vi "BRig_RT_panel_Laser2_v0,902.vi"(7 "input_setValues":bool, 9 "input_dataExp":u16[](array[numeric]), 11 "input_dataLC":u16[](array[numeric])) -> (1 "output_dataExp":u16[](array[numeric]), 3 "output_dataLC":u16[](array[numeric]))   [LabVIEW 2014]
panel:
  out "LaserPulseTrain":cluster{u16[], u16[]}(graph)
  in  "LED_baseline":bool
  in  "Laser_power_step":dbl
  in  "Laser_power_max":dbl
  in  "Laser_power_min":dbl
  in  "Laser_Tshutter":u16=2
  in  "Laser_Freq":u16=10
  in  "Laser_Tpeak":u16=2
  in  "Laser_T":u16
  in  "LC_Sel_PostR_Count":u16
  in  "LC_Sel_PostR_Probability":u16
  in  "LC_Sel_PostR_Block":u16(slide) max=2 step=1 scale=0.0..2.0
  in  "LC_Sel_PostR_OnOff":bool
  in  "LC_Sel_PostR_Tdelay":u16
  in  "LC_Cue_PostR_Count":u16
  in  "LC_Cue_PostR_delayOpt":bool
  in  "LC_Cue_PostR_Probability":u16
  in  "LC_Cue_PostR_Block":u16(slide) max=2 step=1 scale=0.0..2.0
  in  "LC_Cue_PostR_OnOff":bool
  in  "LC_Cue_PostR_Tdelay":u16
  in  "LC_ENL_PostR_delayOpt":bool
  in  "LC_ENL_PostR_Count":u16
  in  "LC_ENL_PostR_Probability":u16 max=100 step=1
  in  "LC_ENL_PostR_Block":u16(slide) max=2 step=1 scale=0.0..2.0
  in  "LC_ENL_PostR_OnOff":bool
  in  "LC_ENL_PostR_Tdelay":u16
  in  "LC_Sel_PreR_Count":u16
  in  "LC_Sel_First_Count":u16
  in  "LC_Sel_PreR_Probability":u16
  in  "LC_Sel_PreR_Block":u16(slide) max=2 step=1 scale=0.0..2.0
  in  "LC_Sel_PreR_OnOff":bool
  in  "LC_Sel_First_Probability":u16
  in  "LC_Sel_First_Block":u16(slide) max=2 step=1 scale=0.0..2.0
  in  "LC_Sel_First_OnOff":bool
  in  "LC_Sel_PreR_Tdelay":u16
  in  "LC_Sel_First_Tdelay":u16
  in  "LC_Cue_PreR_Count":u16
  in  "LC_Cue_First_Count":u16
  in  "LC_Cue_PreR_delayOpt":bool
  in  "LC_ENL_PreR_delayOpt":bool
  in  "LC_ENL_PreR_Count":u16
  in  "LC_ENL_First_Count":u16
  in  "LC_Cue_First_delayOpt":bool
  in  "LC_ENL_First_delayOpt":bool
  in  "LC_Wrong_Probability":u16
  in  "LC_Wrong_Trial":u16(slide) max=2 step=1 scale=0.0..2.0
  in  "LC_Wrong_Block":u16(slide) max=2 step=1 scale=0.0..2.0
  in  "LC_Wrong_OnOff":bool
  in  "LC_Reward_Probability":u16
  in  "LC_Reward_Trial":u16(slide) max=2 step=1 scale=0.0..2.0
  in  "LC_Reward_Block":u16(slide) max=2 step=1 scale=0.0..2.0
  in  "LC_Reward_OnOff":bool
  in  "LC_Cue_PreR_Probability":u16
  in  "LC_Cue_PreR_Block":u16(slide) max=2 step=1 scale=0.0..2.0
  in  "LC_Cue_PreR_OnOff":bool
  in  "LC_Cue_First_Probability":u16
  in  "LC_Cue_First_Block":u16(slide) max=2 step=1 scale=0.0..2.0
  in  "LC_Cue_First_OnOff":bool
  in  "LC_ENL_PreR_Probability":u16 max=100 step=1
  in  "LC_ENL_PreR_Block":u16(slide) max=2 step=1 scale=0.0..2.0
  in  "LC_ENL_PreR_OnOff":bool
  in  "LC_ENL_First_Probability":u16 max=100 step=1
  in  "LC_ENL_First_Block":u16(slide) max=2 step=1 scale=0.0..2.0
  in  "LC_Wrong_Tdelay":u16
  in  "LC_Cue_PreR_Tdelay":u16
  in  "LC_ENL_PreR_Tdelay":u16
  in  "LC_Reward_Tdelay":u16
  in  "LC_Cue_First_Tdelay":u16
  in  "LC_ENL_First_Tdelay":u16
  in  "LC_ENL_First_OnOff":bool
  # "Laser2 Control\n                               On/Off      Block        Probability [%]   Delay [ms]                              Count"
  # "Enforced\nNonLick"
  # "from end"
  # "First\nTrial"
  # "from start"
  # "from end"
  # "PreReward\nTrials"
  # "from start"
  # "from end"
  # "PostReward\nTrials"
  # "from start"
  # "Cue"
  # "from end"
  # "First\nTrial"
  # "from start"
  # "from end"
  # "PreReward\nTrials"
  # "from start"
  # "from end"
  # "PreReward\nTrials"
  # "from start"
  # "Selection"
  # "from start"
  # "First\nTrial"
  # "from start"
  # "PreReward\nTrials"
  # "from start"
  # "PostReward\nTrials"
  # "Laser2 Parameters"
  # "Laser2 Response\n           On/Off      Block           Trial     Probability %  Delay [ms]"
  # "Frequency\n[Hz]"
  # "Selection\nReward"
  # "Timing [ms]\n Duration     Peak Width   Shutter"
  # "Selection\nWrong"
  # "Laser Power [V]\nMin          Max              Step"
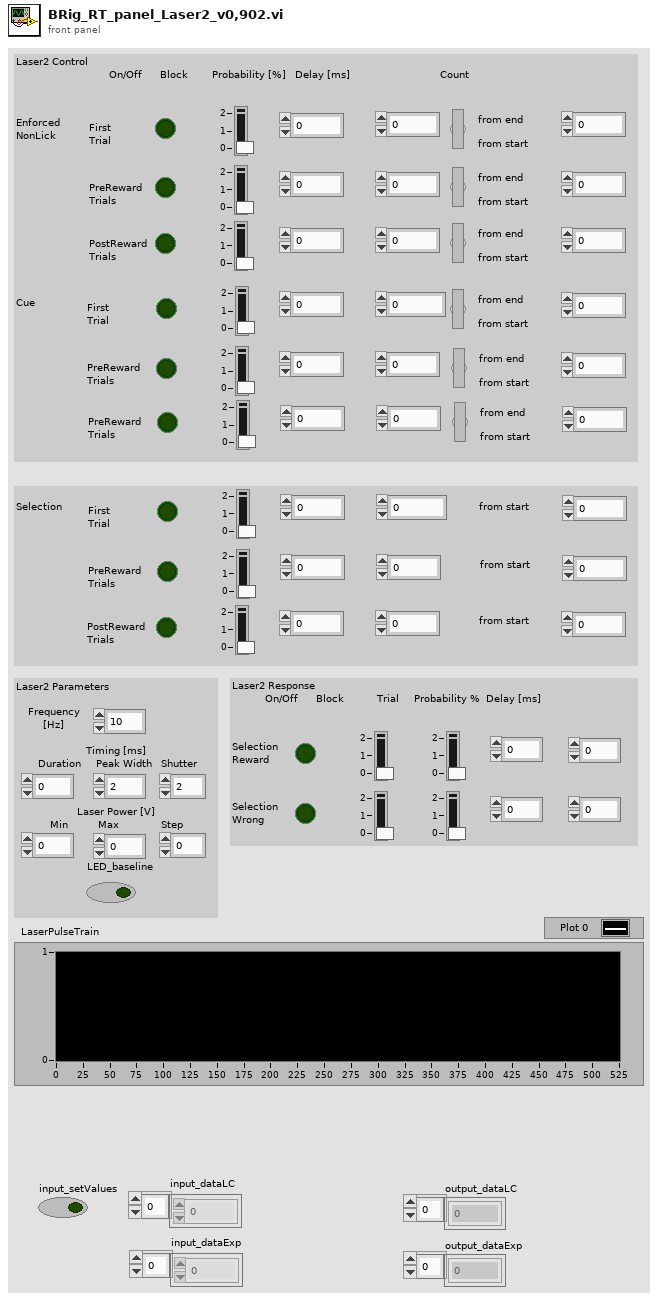
[diagram p1: front panel]
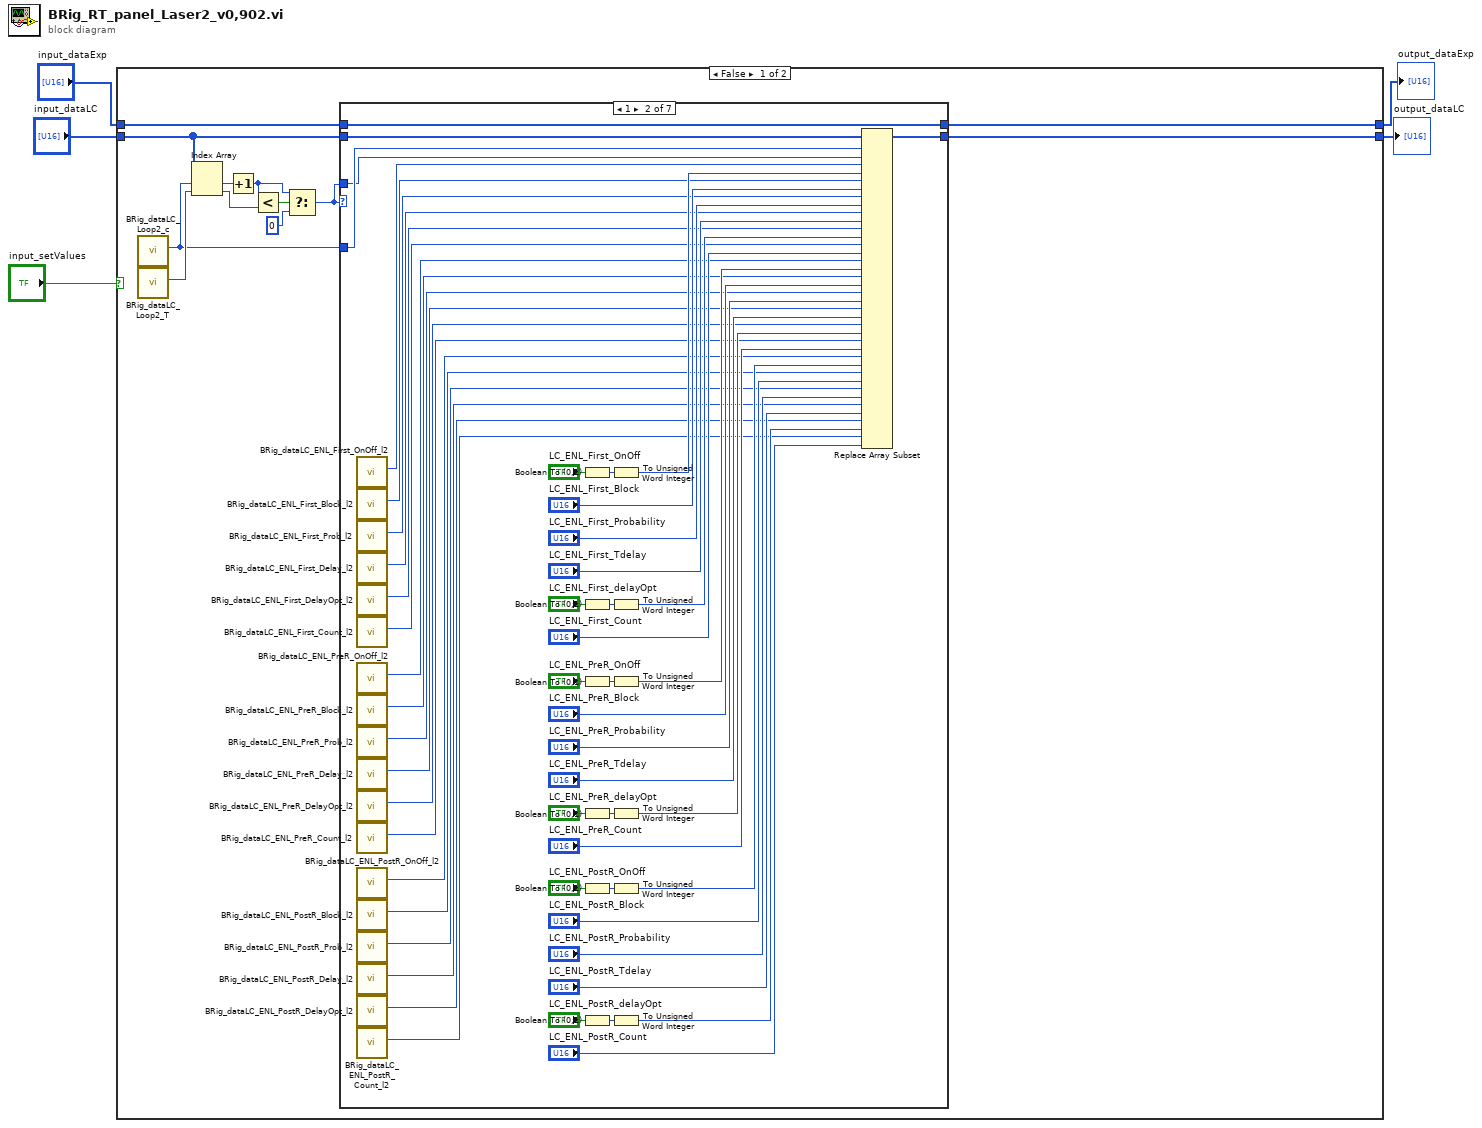
[diagram p0: block diagram]
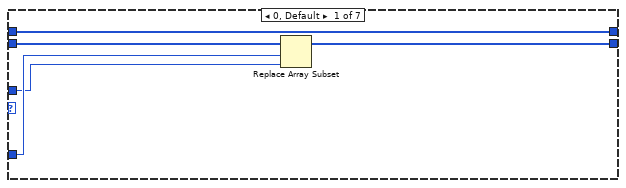
[diagram p2: hidden frame]
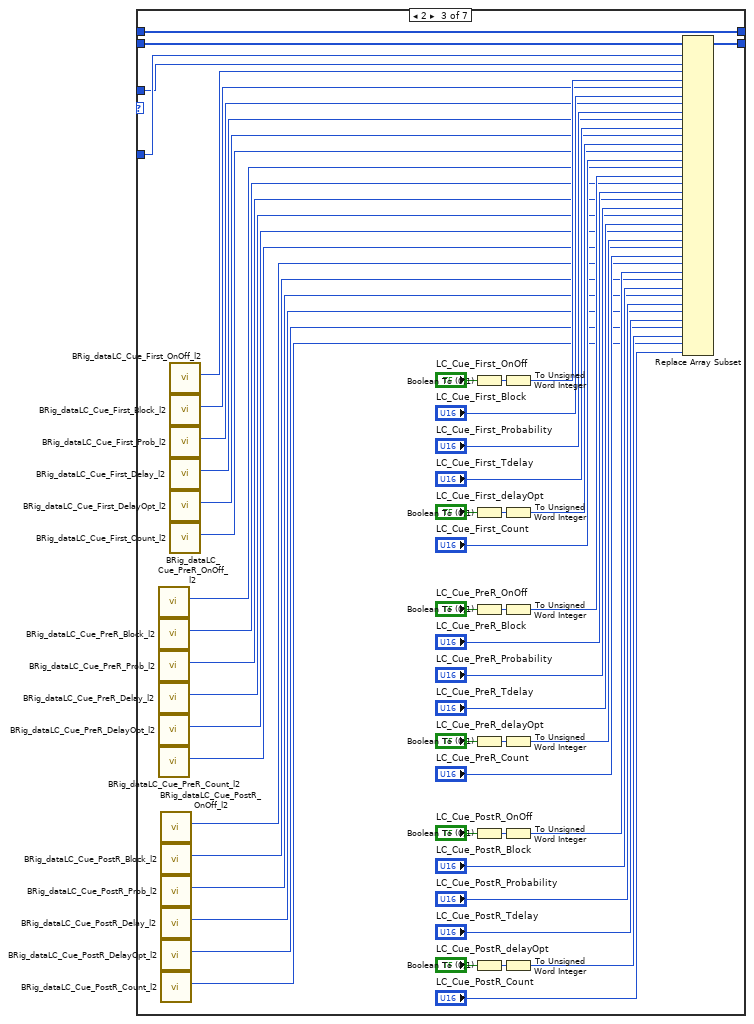
[diagram p3: hidden frame]
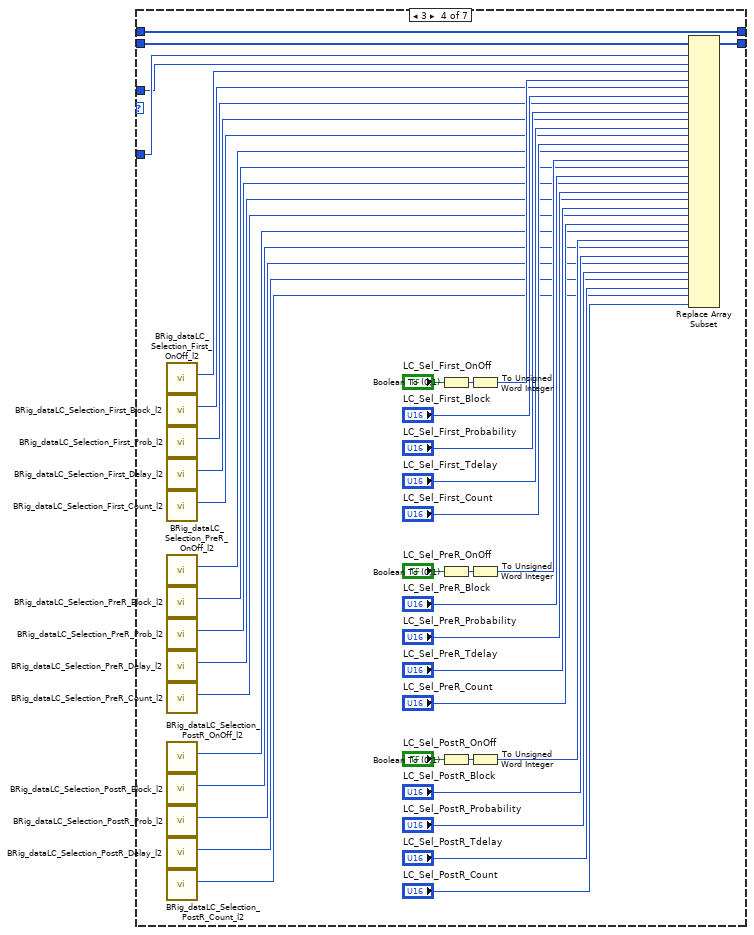
[diagram p4: hidden frame]
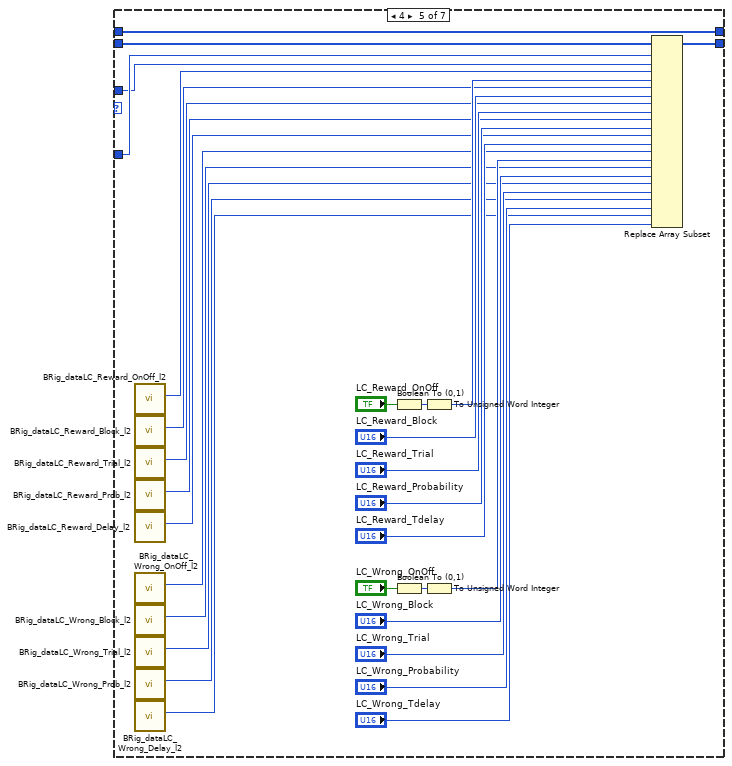
[diagram p5: hidden frame]
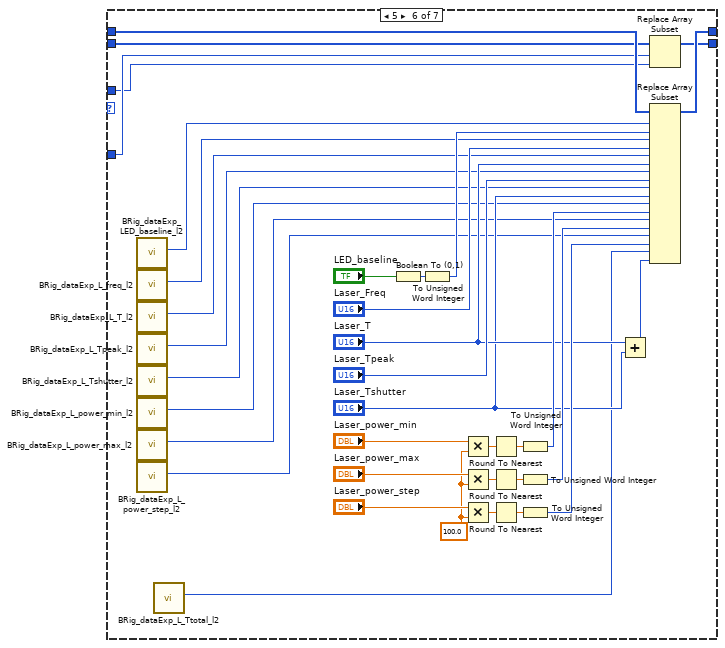
[diagram p6: hidden frame]
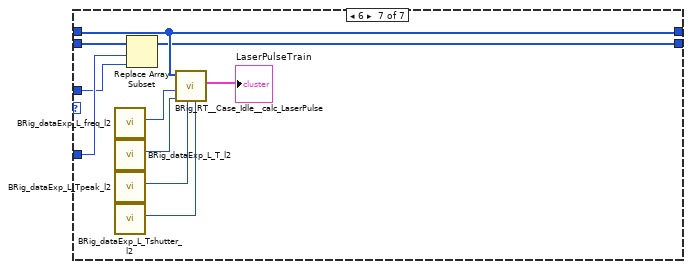
[diagram p7: hidden frame]
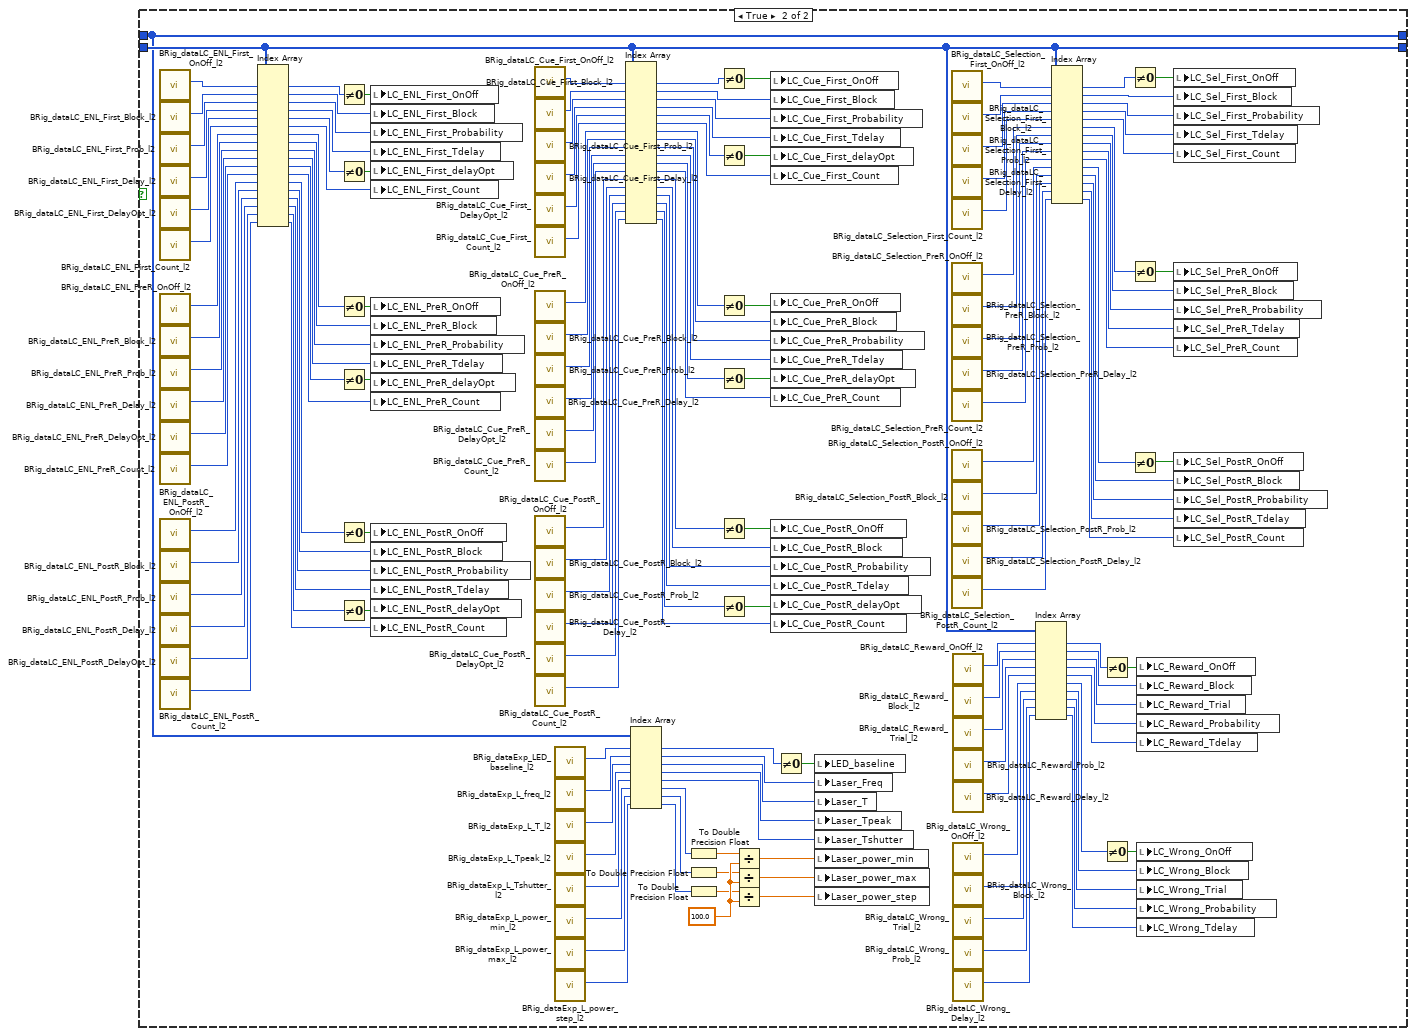
[diagram p8: hidden frame]
diagram:
  n1 = case shown="False" "input_setValues" {
    tunnel: "input_dataLC" -> [w17 w331]
    tunnel: [w11 w331] -> w4
    tunnel: "input_dataExp" -> [w7 w245]
    tunnel: [w6 w245] -> w1
    frame False {
      n2 = call "BRig_dataLC_Loop2_c.vi"() -> ("output_Loop2_c"=w8:i32)  [unwired: 11 in]
      n3 = call "BRig_dataLC_Loop2_T.vi"() -> ("output_Loop2_T"=w9:i32)  [unwired: 11 in]
      n4 = Index Array(array=w17, index #1=w8, index #2=w9) -> (element #1=w16:u16, element #2=w15:u16)
      n5 = Increment(x=w16) -> (x+1=w12:u16)
      n6 = Less?(x=w12, y=w15) -> (x < y?=w14:bool)
      n7 = Select(t=w12, s=w14, f=u16 0) -> (s? t:f=w10:u16)
      n8 = case shown="1" w10 {
        tunnel: w17 -> [w22 w75 w128 w169 w198 w202 w243]
        tunnel: w8 -> [w20 w43 w96 w146 w182 w200 w240]
        tunnel: w10 -> [w19 w42 w95 w145 w181 w199 w239]
        tunnel: [w21 w74 w127 w168 w197 w201 w241] -> w11
        tunnel: w7 -> [w18 w23 w76 w129 w170 w204 w242]
        tunnel: [w18 w23 w76 w129 w170 w203 w242] -> w6
        frame 0, Default {
          n9 = Replace Array Subset(array=w22, new element=w19, index=w20) -> (w21:u16[])
        }
        frame 1 {
          n10 = call "BRig_dataLC_ENL_First_OnOff_l2.vi"() -> ("output_ENL_First_OnOff_l2"=w24:i32)  [unwired: 11 in]
          n11 = call "BRig_dataLC_ENL_First_Block_l2.vi"() -> ("output_ENL_First_Block_l2"=w25:i32)  [unwired: 11 in]
          n12 = call "BRig_dataLC_ENL_First_Prob_l2.vi"() -> ("output_ENL_First_Prob_l2"=w26:i32)  [unwired: 11 in]
          n13 = call "BRig_dataLC_ENL_First_Delay_l2.vi"() -> ("output_ENL_First_Delay_l2"=w27:i32)  [unwired: 11 in]
          n14 = call "BRig_dataLC_ENL_First_DelayOpt_l2.vi"() -> ("output_ENL_First_DelayOpt_l2"=w28:i32)  [unwired: 11 in]
          n15 = call "BRig_dataLC_ENL_First_Count_l2.vi"() -> ("output_ENL_First_Count_l2"=w39:i32)  [unwired: 11 in]
          n16 = call "BRig_dataLC_ENL_PreR_OnOff_l2.vi"() -> ("output_ENL_PreR_OnOff_l2"=w29:i32)  [unwired: 11 in]
          n17 = call "BRig_dataLC_ENL_PreR_Block_l2.vi"() -> ("output_ENL_PreR_Block_l2"=w31:i32)  [unwired: 11 in]
          n18 = call "BRig_dataLC_ENL_PreR_Prob_l2.vi"() -> ("output_ENL_PreR_Prob_l2"=w30:i32)  [unwired: 11 in]
          n19 = call "BRig_dataLC_ENL_PreR_Delay_l2.vi"() -> ("output_ENL_PreR_Delay_l2"=w32:i32)  [unwired: 11 in]
          n20 = call "BRig_dataLC_ENL_PreR_DelayOpt_l2.vi"() -> ("output_ENL_PreR_DelayOpt_l2"=w33:i32)  [unwired: 11 in]
          n21 = call "BRig_dataLC_ENL_PreR_Count_l2.vi"() -> ("output_ENL_PreR_Count_l2"=w40:i32)  [unwired: 11 in]
          n22 = call "BRig_dataLC_ENL_PostR_OnOff_l2.vi"() -> ("output_ENL_PostR_OnOff_l2"=w34:i32)  [unwired: 11 in]
          n23 = call "BRig_dataLC_ENL_PostR_Block_l2.vi"() -> ("output_ENL_PostR_Block_l2"=w35:i32)  [unwired: 11 in]
          n24 = call "BRig_dataLC_ENL_PostR_Prob_l2.vi"() -> ("output_ENL_PostR_Prob_l2"=w36:i32)  [unwired: 11 in]
          n25 = call "BRig_dataLC_ENL_PostR_Delay_l2.vi"() -> ("output_ENL_PostR_Delay_l2"=w37:i32)  [unwired: 11 in]
          n26 = call "BRig_dataLC_ENL_PostR_DelayOpt_l2.vi"() -> ("output_ENL_PostR_DelayOpt_l2"=w38:i32)  [unwired: 11 in]
          n27 = call "BRig_dataLC_ENL_PostR_Count_l2.vi"() -> ("output_ENL_PostR_Count_l2"=w41:i32)  [unwired: 11 in]
          n28 = Boolean To (0,1)(Boolean="LC_ENL_First_OnOff") -> (0, 1=w72:i16)
          n29 = Boolean To (0,1)(Boolean="LC_ENL_First_delayOpt") -> (0, 1=w71:i16)
          n30 = Boolean To (0,1)(Boolean="LC_ENL_PreR_OnOff") -> (0, 1=w69:i16)
          n31 = Boolean To (0,1)(Boolean="LC_ENL_PreR_delayOpt") -> (0, 1=w67:i16)
          n32 = Boolean To (0,1)(Boolean="LC_ENL_PostR_OnOff") -> (0, 1=w65:i16)
          n33 = Boolean To (0,1)(Boolean="LC_ENL_PostR_delayOpt") -> (0, 1=w63:i16)
          n34 = To Unsigned Word Integer(number=w72) -> (unsigned 16bit integer=w61:u16)
          n35 = To Unsigned Word Integer(number=w71) -> (unsigned 16bit integer=w57:u16)
          n36 = To Unsigned Word Integer(number=w69) -> (unsigned 16bit integer=w55:u16)
          n37 = To Unsigned Word Integer(number=w67) -> (unsigned 16bit integer=w51:u16)
          n38 = To Unsigned Word Integer(number=w65) -> (unsigned 16bit integer=w49:u16)
          n39 = To Unsigned Word Integer(number=w63) -> (unsigned 16bit integer=w45:u16)
          n40 = Replace Array Subset(array=w75, new element #1=w42, index #1=w43, new element #2=w61, index #2=w24, new element #3="LC_ENL_First_Block", index #3=w25, new element #4="LC_ENL_First_Probability", index #4=w26, new element #5="LC_ENL_First_Tdelay", index #5=w27, new element #6=w57, index #6=w28, new element #7="LC_ENL_First_Count", index #7=w39, new element #8=w55, index #8=w29, new element #9="LC_ENL_PreR_Block", index #9=w31, new element #10="LC_ENL_PreR_Probability", index #10=w30, new element #11="LC_ENL_PreR_Tdelay", index #11=w32, new element #12=w51, index #12=w33, new element #13="LC_ENL_PreR_Count", index #13=w40, new element #14=w49, index #14=w34, new element #15="LC_ENL_PostR_Block", index #15=w35, new element #16="LC_ENL_PostR_Probability", index #16=w36, new element #17="LC_ENL_PostR_Tdelay", index #17=w37, new element #18=w45, index #18=w38, new element #19="LC_ENL_PostR_Count", index #19=w41) -> (w74:u16[])
        }
        frame 2 {
          n41 = call "BRig_dataLC_Cue_PreR_OnOff_l2.vi"() -> ("output_Cue_PreR_OnOff_l2"=w83:i32)  [unwired: 11 in]
          n42 = call "BRig_dataLC_Cue_PreR_Block_l2.vi"() -> ("output_Cue_PreR_Block_l2"=w84:i32)  [unwired: 11 in]
          n43 = call "BRig_dataLC_Cue_PreR_Prob_l2.vi"() -> ("output_Cue_PreR_Prob_l2"=w85:i32)  [unwired: 11 in]
          n44 = call "BRig_dataLC_Cue_PreR_Delay_l2.vi"() -> ("output_Cue_PreR_Delay_l2"=w86:i32)  [unwired: 11 in]
          n45 = call "BRig_dataLC_Cue_PreR_DelayOpt_l2.vi"() -> ("output_Cue_PreR_DelayOpt_l2"=w87:i32)  [unwired: 11 in]
          n46 = call "BRig_dataLC_Cue_PreR_Count_l2.vi"() -> ("output_Cue_PreR_Count_l2"=w88:i32)  [unwired: 11 in]
          n47 = call "BRig_dataLC_Cue_PostR_OnOff_l2.vi"() -> ("output_Cue_PostR_OnOff_l2"=w82:i32)  [unwired: 11 in]
          n48 = call "BRig_dataLC_Cue_PostR_Block_l2.vi"() -> ("output_Cue_PostR_Block_l2"=w77:i32)  [unwired: 11 in]
          n49 = call "BRig_dataLC_Cue_PostR_Prob_l2.vi"() -> ("output_Cue_PostR_Prob_l2"=w78:i32)  [unwired: 11 in]
          n50 = call "BRig_dataLC_Cue_PostR_Delay_l2.vi"() -> ("output_Cue_PostR_Delay_l2"=w79:i32)  [unwired: 11 in]
          n51 = call "BRig_dataLC_Cue_PostR_DelayOpt_l2.vi"() -> ("output_Cue_PostR_DelayOpt_l2"=w80:i32)  [unwired: 11 in]
          n52 = call "BRig_dataLC_Cue_PostR_Count_l2.vi"() -> ("output_Cue_PostR_Count_l2"=w81:i32)  [unwired: 11 in]
          n53 = call "BRig_dataLC_Cue_First_OnOff_l2.vi"() -> ("output_Cue_First_OnOff_l2"=w89:i32)  [unwired: 11 in]
          n54 = call "BRig_dataLC_Cue_First_Block_l2.vi"() -> ("output_Cue_First_Block_l2"=w90:i32)  [unwired: 11 in]
          n55 = call "BRig_dataLC_Cue_First_Prob_l2.vi"() -> ("output_Cue_First_Prob_l2"=w91:i32)  [unwired: 11 in]
          n56 = call "BRig_dataLC_Cue_First_Delay_l2.vi"() -> ("output_Cue_First_Delay_l2"=w92:i32)  [unwired: 11 in]
          n57 = call "BRig_dataLC_Cue_First_DelayOpt_l2.vi"() -> ("output_Cue_First_DelayOpt_l2"=w93:i32)  [unwired: 11 in]
          n58 = call "BRig_dataLC_Cue_First_Count_l2.vi"() -> ("output_Cue_First_Count_l2"=w94:i32)  [unwired: 11 in]
          n59 = Boolean To (0,1)(Boolean="LC_Cue_First_OnOff") -> (0, 1=w120:i16)
          n60 = Boolean To (0,1)(Boolean="LC_Cue_First_delayOpt") -> (0, 1=w119:i16)
          n61 = Boolean To (0,1)(Boolean="LC_Cue_PreR_OnOff") -> (0, 1=w118:i16)
          n62 = Boolean To (0,1)(Boolean="LC_Cue_PreR_delayOpt") -> (0, 1=w117:i16)
          n63 = Boolean To (0,1)(Boolean="LC_Cue_PostR_OnOff") -> (0, 1=w116:i16)
          n64 = Boolean To (0,1)(Boolean="LC_Cue_PostR_delayOpt") -> (0, 1=w115:i16)
          n65 = To Unsigned Word Integer(number=w120) -> (unsigned 16bit integer=w114:u16)
          n66 = To Unsigned Word Integer(number=w119) -> (unsigned 16bit integer=w110:u16)
          n67 = To Unsigned Word Integer(number=w118) -> (unsigned 16bit integer=w108:u16)
          n68 = To Unsigned Word Integer(number=w117) -> (unsigned 16bit integer=w104:u16)
          n69 = To Unsigned Word Integer(number=w116) -> (unsigned 16bit integer=w102:u16)
          n70 = To Unsigned Word Integer(number=w115) -> (unsigned 16bit integer=w98:u16)
          n71 = Replace Array Subset(array=w128, new element #1=w95, index #1=w96, new element #2=w114, index #2=w89, new element #3="LC_Cue_First_Block", index #3=w90, new element #4="LC_Cue_First_Probability", index #4=w91, new element #5="LC_Cue_First_Tdelay", index #5=w92, new element #6=w110, index #6=w93, new element #7="LC_Cue_First_Count", index #7=w94, new element #8=w108, index #8=w83, new element #9="LC_Cue_PreR_Block", index #9=w84, new element #10="LC_Cue_PreR_Probability", index #10=w85, new element #11="LC_Cue_PreR_Tdelay", index #11=w86, new element #12=w104, index #12=w87, new element #13="LC_Cue_PreR_Count", index #13=w88, new element #14=w102, index #14=w82, new element #15="LC_Cue_PostR_Block", index #15=w77, new element #16="LC_Cue_PostR_Probability", index #16=w78, new element #17="LC_Cue_PostR_Tdelay", index #17=w79, new element #18=w98, index #18=w80, new element #19="LC_Cue_PostR_Count", index #19=w81) -> (w127:u16[])
        }
        frame 3 {
          n72 = call "BRig_dataLC_Selection_First_OnOff_l2.vi"() -> ("output_Selection_First_OnOff_l2"=w130:i32)  [unwired: 11 in]
          n73 = call "BRig_dataLC_Selection_First_Block_l2.vi"() -> ("output_Selection_First_Block_l2"=w131:i32)  [unwired: 11 in]
          n74 = call "BRig_dataLC_Selection_First_Prob_l2.vi"() -> ("output_Selection_First_Prob_l2"=w132:i32)  [unwired: 11 in]
          n75 = call "BRig_dataLC_Selection_First_Delay_l2.vi"() -> ("output_Selection_First_Delay_l2"=w133:i32)  [unwired: 11 in]
          n76 = call "BRig_dataLC_Selection_First_Count_l2.vi"() -> ("output_Selection_First_Count_l2"=w134:i32)  [unwired: 11 in]
          n77 = call "BRig_dataLC_Selection_PreR_OnOff_l2.vi"() -> ("output_Selection_PreR_OnOff_l2"=w135:i32)  [unwired: 11 in]
          n78 = call "BRig_dataLC_Selection_PreR_Block_l2.vi"() -> ("output_Selection_PreR_Block_l2"=w136:i32)  [unwired: 11 in]
          n79 = call "BRig_dataLC_Selection_PreR_Prob_l2.vi"() -> ("output_Selection_PreR_Prob_l2"=w137:i32)  [unwired: 11 in]
          n80 = call "BRig_dataLC_Selection_PreR_Delay_l2.vi"() -> ("output_Selection_PreR_Delay_l2"=w138:i32)  [unwired: 11 in]
          n81 = call "BRig_dataLC_Selection_PreR_Count_l2.vi"() -> ("output_Selection_PreR_Count_l2"=w139:i32)  [unwired: 11 in]
          n82 = call "BRig_dataLC_Selection_PostR_OnOff_l2.vi"() -> ("output_Selection_PostR_OnOff_l2"=w140:i32)  [unwired: 11 in]
          n83 = call "BRig_dataLC_Selection_PostR_Block_l2.vi"() -> ("output_Selection_PostR_Block_l2"=w141:i32)  [unwired: 11 in]
          n84 = call "BRig_dataLC_Selection_PostR_Prob_l2.vi"() -> ("output_Selection_PostR_Prob_l2"=w142:i32)  [unwired: 11 in]
          n85 = call "BRig_dataLC_Selection_PostR_Delay_l2.vi"() -> ("output_Selection_PostR_Delay_l2"=w143:i32)  [unwired: 11 in]
          n86 = call "BRig_dataLC_Selection_PostR_Count_l2.vi"() -> ("output_Selection_PostR_Count_l2"=w144:i32)  [unwired: 11 in]
          n87 = Boolean To (0,1)(Boolean="LC_Sel_First_OnOff") -> (0, 1=w164:i16)
          n88 = Boolean To (0,1)(Boolean="LC_Sel_PreR_OnOff") -> (0, 1=w163:i16)
          n89 = Boolean To (0,1)(Boolean="LC_Sel_PostR_OnOff") -> (0, 1=w162:i16)
          n90 = To Unsigned Word Integer(number=w164) -> (unsigned 16bit integer=w161:u16)
          n91 = To Unsigned Word Integer(number=w163) -> (unsigned 16bit integer=w156:u16)
          n92 = To Unsigned Word Integer(number=w162) -> (unsigned 16bit integer=w151:u16)
          n93 = Replace Array Subset(array=w169, new element #1=w145, index #1=w146, new element #2=w161, index #2=w130, new element #3="LC_Sel_First_Block", index #3=w131, new element #4="LC_Sel_First_Probability", index #4=w132, new element #5="LC_Sel_First_Tdelay", index #5=w133, new element #6="LC_Sel_First_Count", index #6=w134, new element #7=w156, index #7=w135, new element #8="LC_Sel_PreR_Block", index #8=w136, new element #9="LC_Sel_PreR_Probability", index #9=w137, new element #10="LC_Sel_PreR_Tdelay", index #10=w138, new element #11="LC_Sel_PreR_Count", index #11=w139, new element #12=w151, index #12=w140, new element #13="LC_Sel_PostR_Block", index #13=w141, new element #14="LC_Sel_PostR_Probability", index #14=w142, new element #15="LC_Sel_PostR_Tdelay", index #15=w143, new element #16="LC_Sel_PostR_Count", index #16=w144) -> (w168:u16[])
        }
        frame 4 {
          n94 = call "BRig_dataLC_Reward_OnOff_l2.vi"() -> ("output_Reward_OnOff_l2"=w171:i32)  [unwired: 11 in]
          n95 = call "BRig_dataLC_Reward_Block_l2.vi"() -> ("output_Reward_Block_l2"=w172:i32)  [unwired: 11 in]
          n96 = call "BRig_dataLC_Reward_Trial_l2.vi"() -> ("output_Reward_Trial_l2"=w173:i32)  [unwired: 11 in]
          n97 = call "BRig_dataLC_Reward_Prob_l2.vi"() -> ("output_Reward_Prob_l2"=w174:i32)  [unwired: 11 in]
          n98 = call "BRig_dataLC_Reward_Delay_l2.vi"() -> ("output_Reward_Delay_l2"=w175:i32)  [unwired: 11 in]
          n99 = call "BRig_dataLC_Wrong_OnOff_l2.vi"() -> ("output_Wrong_OnOff_l2"=w176:i32)  [unwired: 11 in]
          n100 = call "BRig_dataLC_Wrong_Block_l2.vi"() -> ("output_Wrong_Block_l2"=w177:i32)  [unwired: 11 in]
          n101 = call "BRig_dataLC_Wrong_Trial_l2.vi"() -> ("output_Wrong_Trial_l2"=w178:i32)  [unwired: 11 in]
          n102 = call "BRig_dataLC_Wrong_Prob_l2.vi"() -> ("output_Wrong_Prob_l2"=w179:i32)  [unwired: 11 in]
          n103 = call "BRig_dataLC_Wrong_Delay_l2.vi"() -> ("output_Wrong_Delay_l2"=w180:i32)  [unwired: 11 in]
          n104 = Boolean To (0,1)(Boolean="LC_Reward_OnOff") -> (0, 1=w194:i16)
          n105 = Boolean To (0,1)(Boolean="LC_Wrong_OnOff") -> (0, 1=w193:i16)
          n106 = To Unsigned Word Integer(number=w194) -> (unsigned 16bit integer=w192:u16)
          n107 = To Unsigned Word Integer(number=w193) -> (unsigned 16bit integer=w187:u16)
          n108 = Replace Array Subset(array=w198, new element #1=w181, index #1=w182, new element #2=w192, index #2=w171, new element #3="LC_Reward_Block", index #3=w172, new element #4="LC_Reward_Trial", index #4=w173, new element #5="LC_Reward_Probability", index #5=w174, new element #6="LC_Reward_Tdelay", index #6=w175, new element #7=w187, index #7=w176, new element #8="LC_Wrong_Block", index #8=w177, new element #9="LC_Wrong_Trial", index #9=w178, new element #10="LC_Wrong_Probability", index #10=w179, new element #11="LC_Wrong_Tdelay", index #11=w180) -> (w197:u16[])
        }
        frame 5 {
          w222 = 100.0 ("y")
          n109 = call "BRig_dataExp_LED_baseline_l2.vi"() -> ("output_LED_baseline_l2"=w212:i32)  [unwired: 11 in]
          n110 = call "BRig_dataExp_L_freq_l2.vi"() -> ("output_L_freq_l2"=w211:i32)  [unwired: 11 in]
          n111 = call "BRig_dataExp_L_T_l2.vi"() -> ("output_L_T_l2"=w210:i32)  [unwired: 11 in]
          n112 = call "BRig_dataExp_L_Tpeak_l2.vi"() -> ("output_L_Tpeak_l2"=w209:i32)  [unwired: 11 in]
          n113 = call "BRig_dataExp_L_Tshutter_l2.vi"() -> ("output_L_Tshutter_l2"=w208:i32)  [unwired: 11 in]
          n114 = call "BRig_dataExp_L_power_min_l2.vi"() -> ("output_L_power_min_l2"=w207:i32)  [unwired: 11 in]
          n115 = call "BRig_dataExp_L_power_max_l2.vi"() -> ("output_L_power_max_l2"=w206:i32)  [unwired: 11 in]
          n116 = call "BRig_dataExp_L_power_step_l2.vi"() -> ("output_L_power_step_l2"=w205:i32)  [unwired: 11 in]
          n117 = call "BRig_dataExp_L_Ttotal_l2.vi"() -> ("output_L_Ttotal_l2"=w213:i32)  [unwired: 11 in]
          n118 = Boolean To (0,1)(Boolean="LED_baseline") -> (0, 1=w234:i16)
          n119 = To Unsigned Word Integer(number=w234) -> (unsigned 16bit integer=w232:u16)
          n120 = Multiply(x="Laser_power_min", y=w222) -> (x*y=w226:dbl)
          n121 = Multiply(x="Laser_power_max", y=w222) -> (x*y=w228:dbl)
          n122 = Multiply(x="Laser_power_step", y=w222) -> (x*y=w231:dbl)
          n123 = Round To Nearest(number=w226) -> (nearest integer value=w225:dbl)
          n124 = Round To Nearest(number=w228) -> (nearest integer value=w227:dbl)
          n125 = Round To Nearest(number=w231) -> (nearest integer value=w230:dbl)
          n126 = To Unsigned Word Integer(number=w225) -> (unsigned 16bit integer=w219:u16)
          n127 = To Unsigned Word Integer(number=w227) -> (unsigned 16bit integer=w220:u16)
          n128 = To Unsigned Word Integer(number=w230) -> (unsigned 16bit integer=w221:u16)
          n129 = Add(x="Laser_T", y="Laser_Tshutter") -> (x+y=w214:u16)
          n130 = Replace Array Subset(array=w202, new element=w199, index=w200) -> (w201:u16[])
          n131 = Replace Array Subset(array=w204, new element #1=w232, index #1=w212, new element #2="Laser_Freq", index #2=w211, new element #3="Laser_T", index #3=w210, new element #4="Laser_Tpeak", index #4=w209, new element #5="Laser_Tshutter", index #5=w208, new element #6=w219, index #6=w207, new element #7=w220, index #7=w206, new element #8=w221, index #8=w205, new element #9=w214, index #9=w213) -> (w203:u16[])
        }
        frame 6 {
          n132 = call "BRig_dataExp_L_freq_l2.vi"() -> ("output_L_freq_l2"=w237:i32)  [unwired: 11 in]
          n133 = call "BRig_dataExp_L_T_l2.vi"() -> ("output_L_T_l2"=w238:i32)  [unwired: 11 in]
          n134 = call "BRig_dataExp_L_Tpeak_l2.vi"() -> ("output_L_Tpeak_l2"=w236:i32)  [unwired: 11 in]
          n135 = call "BRig_dataExp_L_Tshutter_l2.vi"() -> ("output_L_Tshutter_l2"=w235:i32)  [unwired: 11 in]
          n136 = Replace Array Subset(array=w243, new element=w239, index=w240) -> (w241:u16[])
          n137 = call "BRig_RT__Case_Idle__calc_LaserPulse.vi"("input_dataExp_L_Tshutter"=w235, "input_dataExp_L_Tpeak"=w236, "input_dataExp_L_T"=w238, "input_dataExp_L_freq"=w237, "input_dataExp"=w242) -> ("output_cluster"=→"LaserPulseTrain":cluster{u16[], u16[]})  [unwired: 6 in]
        }
      }
    }
    frame True {
      w317 = 100.0 ("y")
      n138 = call "BRig_dataLC_ENL_First_OnOff_l2.vi"() -> ("output_ENL_First_OnOff_l2"=w297:i32)  [unwired: 11 in]
      n139 = call "BRig_dataLC_ENL_First_Block_l2.vi"() -> ("output_ENL_First_Block_l2"=w298:i32)  [unwired: 11 in]
      n140 = call "BRig_dataLC_ENL_First_Prob_l2.vi"() -> ("output_ENL_First_Prob_l2"=w299:i32)  [unwired: 11 in]
      n141 = call "BRig_dataLC_ENL_First_Delay_l2.vi"() -> ("output_ENL_First_Delay_l2"=w300:i32)  [unwired: 11 in]
      n142 = call "BRig_dataLC_ENL_First_DelayOpt_l2.vi"() -> ("output_ENL_First_DelayOpt_l2"=w301:i32)  [unwired: 11 in]
      n143 = call "BRig_dataLC_ENL_First_Count_l2.vi"() -> ("output_ENL_First_Count_l2"=w312:i32)  [unwired: 11 in]
      n144 = call "BRig_dataLC_ENL_PreR_OnOff_l2.vi"() -> ("output_ENL_PreR_OnOff_l2"=w302:i32)  [unwired: 11 in]
      n145 = call "BRig_dataLC_ENL_PreR_Block_l2.vi"() -> ("output_ENL_PreR_Block_l2"=w303:i32)  [unwired: 11 in]
      n146 = call "BRig_dataLC_ENL_PreR_Prob_l2.vi"() -> ("output_ENL_PreR_Prob_l2"=w304:i32)  [unwired: 11 in]
      n147 = call "BRig_dataLC_ENL_PreR_Delay_l2.vi"() -> ("output_ENL_PreR_Delay_l2"=w305:i32)  [unwired: 11 in]
      n148 = call "BRig_dataLC_ENL_PreR_DelayOpt_l2.vi"() -> ("output_ENL_PreR_DelayOpt_l2"=w306:i32)  [unwired: 11 in]
      n149 = call "BRig_dataLC_ENL_PreR_Count_l2.vi"() -> ("output_ENL_PreR_Count_l2"=w313:i32)  [unwired: 11 in]
      n150 = call "BRig_dataLC_ENL_PostR_OnOff_l2.vi"() -> ("output_ENL_PostR_OnOff_l2"=w307:i32)  [unwired: 11 in]
      n151 = call "BRig_dataLC_ENL_PostR_Block_l2.vi"() -> ("output_ENL_PostR_Block_l2"=w308:i32)  [unwired: 11 in]
      n152 = call "BRig_dataLC_ENL_PostR_Prob_l2.vi"() -> ("output_ENL_PostR_Prob_l2"=w309:i32)  [unwired: 11 in]
      n153 = call "BRig_dataLC_ENL_PostR_Delay_l2.vi"() -> ("output_ENL_PostR_Delay_l2"=w310:i32)  [unwired: 11 in]
      n154 = call "BRig_dataLC_ENL_PostR_DelayOpt_l2.vi"() -> ("output_ENL_PostR_DelayOpt_l2"=w311:i32)  [unwired: 11 in]
      n155 = call "BRig_dataLC_ENL_PostR_Count_l2.vi"() -> ("output_ENL_PostR_Count_l2"=w314:i32)  [unwired: 11 in]
      n156 = Index Array(array=w331, index #1=w297, index #2=w298, index #3=w299, index #4=w300, index #5=w301, index #6=w312, index #7=w302, index #8=w303, index #9=w304, index #10=w305, index #11=w306, index #12=w313, index #13=w307, index #14=w308, index #15=w309, index #16=w310, index #17=w311, index #18=w314) -> (element #1=w403:u16, element #2=w402:u16, element #3=w401:u16, element #4=w400:u16, element #5=w399:u16, element #6=w398:u16, element #7=w397:u16, element #8=w396:u16, element #9=w395:u16, element #10=w394:u16, element #11=w393:u16, element #12=w392:u16, element #13=w391:u16, element #14=w390:u16, element #15=w389:u16, element #16=w388:u16, element #17=w387:u16, element #18=w386:u16)
      n157 = Not Equal To 0?(x=w403) -> (x != 0?=w409:bool)
      n158 = Not Equal To 0?(x=w399) -> (x != 0?=w408:bool)
      n159 = Not Equal To 0?(x=w397) -> (x != 0?=w407:bool)
      n160 = Not Equal To 0?(x=w393) -> (x != 0?=w406:bool)
      n161 = Not Equal To 0?(x=w391) -> (x != 0?=w405:bool)
      n162 = Not Equal To 0?(x=w387) -> (x != 0?=w404:bool)
      n163 = local write "LC_ENL_First_OnOff"(w409) -> ()
      n164 = local write "LC_ENL_First_Block"(w402) -> ()
      n165 = local write "LC_ENL_First_Probability"(w401) -> ()
      n166 = local write "LC_ENL_First_Tdelay"(w400) -> ()
      n167 = local write "LC_ENL_First_delayOpt"(w408) -> ()
      n168 = local write "LC_ENL_First_Count"(w398) -> ()
      n169 = local write "LC_ENL_PreR_OnOff"(w407) -> ()
      n170 = local write "LC_ENL_PreR_Block"(w396) -> ()
      n171 = local write "LC_ENL_PreR_Probability"(w395) -> ()
      n172 = local write "LC_ENL_PreR_Tdelay"(w394) -> ()
      n173 = local write "LC_ENL_PreR_delayOpt"(w406) -> ()
      n174 = local write "LC_ENL_PreR_Count"(w392) -> ()
      n175 = local write "LC_ENL_PostR_OnOff"(w405) -> ()
      n176 = local write "LC_ENL_PostR_Block"(w390) -> ()
      n177 = local write "LC_ENL_PostR_Probability"(w389) -> ()
      n178 = local write "LC_ENL_PostR_Tdelay"(w388) -> ()
      n179 = local write "LC_ENL_PostR_delayOpt"(w404) -> ()
      n180 = local write "LC_ENL_PostR_Count"(w386) -> ()
      n181 = call "BRig_dataLC_Cue_First_OnOff_l2.vi"() -> ("output_Cue_First_OnOff_l2"=w291:i32)  [unwired: 11 in]
      n182 = call "BRig_dataLC_Cue_First_Block_l2.vi"() -> ("output_Cue_First_Block_l2"=w292:i32)  [unwired: 11 in]
      n183 = call "BRig_dataLC_Cue_First_Prob_l2.vi"() -> ("output_Cue_First_Prob_l2"=w293:i32)  [unwired: 11 in]
      n184 = call "BRig_dataLC_Cue_First_Delay_l2.vi"() -> ("output_Cue_First_Delay_l2"=w294:i32)  [unwired: 11 in]
      n185 = call "BRig_dataLC_Cue_First_DelayOpt_l2.vi"() -> ("output_Cue_First_DelayOpt_l2"=w295:i32)  [unwired: 11 in]
      n186 = call "BRig_dataLC_Cue_First_Count_l2.vi"() -> ("output_Cue_First_Count_l2"=w296:i32)  [unwired: 11 in]
      n187 = call "BRig_dataLC_Cue_PreR_OnOff_l2.vi"() -> ("output_Cue_PreR_OnOff_l2"=w256:i32)  [unwired: 11 in]
      n188 = call "BRig_dataLC_Cue_PreR_Block_l2.vi"() -> ("output_Cue_PreR_Block_l2"=w255:i32)  [unwired: 11 in]
      n189 = call "BRig_dataLC_Cue_PreR_Prob_l2.vi"() -> ("output_Cue_PreR_Prob_l2"=w254:i32)  [unwired: 11 in]
      n190 = call "BRig_dataLC_Cue_PreR_Delay_l2.vi"() -> ("output_Cue_PreR_Delay_l2"=w253:i32)  [unwired: 11 in]
      n191 = call "BRig_dataLC_Cue_PreR_DelayOpt_l2.vi"() -> ("output_Cue_PreR_DelayOpt_l2"=w252:i32)  [unwired: 11 in]
      n192 = call "BRig_dataLC_Cue_PreR_Count_l2.vi"() -> ("output_Cue_PreR_Count_l2"=w257:i32)  [unwired: 11 in]
      n193 = call "BRig_dataLC_Cue_PostR_OnOff_l2.vi"() -> ("output_Cue_PostR_OnOff_l2"=w250:i32)  [unwired: 11 in]
      n194 = call "BRig_dataLC_Cue_PostR_Block_l2.vi"() -> ("output_Cue_PostR_Block_l2"=w249:i32)  [unwired: 11 in]
      n195 = call "BRig_dataLC_Cue_PostR_Prob_l2.vi"() -> ("output_Cue_PostR_Prob_l2"=w248:i32)  [unwired: 11 in]
      n196 = call "BRig_dataLC_Cue_PostR_Delay_l2.vi"() -> ("output_Cue_PostR_Delay_l2"=w247:i32)  [unwired: 11 in]
      n197 = call "BRig_dataLC_Cue_PostR_DelayOpt_l2.vi"() -> ("output_Cue_PostR_DelayOpt_l2"=w246:i32)  [unwired: 11 in]
      n198 = call "BRig_dataLC_Cue_PostR_Count_l2.vi"() -> ("output_Cue_PostR_Count_l2"=w251:i32)  [unwired: 11 in]
      n199 = call "BRig_dataExp_LED_baseline_l2.vi"() -> ("output_LED_baseline_l2"=w268:i32)  [unwired: 11 in]
      n200 = call "BRig_dataExp_L_freq_l2.vi"() -> ("output_L_freq_l2"=w269:i32)  [unwired: 11 in]
      n201 = call "BRig_dataExp_L_T_l2.vi"() -> ("output_L_T_l2"=w270:i32)  [unwired: 11 in]
      n202 = call "BRig_dataExp_L_Tpeak_l2.vi"() -> ("output_L_Tpeak_l2"=w271:i32)  [unwired: 11 in]
      n203 = call "BRig_dataExp_L_Tshutter_l2.vi"() -> ("output_L_Tshutter_l2"=w272:i32)  [unwired: 11 in]
      n204 = call "BRig_dataExp_L_power_min_l2.vi"() -> ("output_L_power_min_l2"=w273:i32)  [unwired: 11 in]
      n205 = call "BRig_dataExp_L_power_max_l2.vi"() -> ("output_L_power_max_l2"=w274:i32)  [unwired: 11 in]
      n206 = call "BRig_dataExp_L_power_step_l2.vi"() -> ("output_L_power_step_l2"=w275:i32)  [unwired: 11 in]
      n207 = Index Array(array=w331, index #1=w291, index #2=w292, index #3=w293, index #4=w294, index #5=w295, index #6=w296, index #7=w256, index #8=w255, index #9=w254, index #10=w253, index #11=w252, index #12=w257, index #13=w250, index #14=w249, index #15=w248, index #16=w247, index #17=w246, index #18=w251) -> (element #1=w379:u16, element #2=w378:u16, element #3=w377:u16, element #4=w376:u16, element #5=w375:u16, element #6=w374:u16, element #7=w373:u16, element #8=w372:u16, element #9=w371:u16, element #10=w370:u16, element #11=w369:u16, element #12=w368:u16, element #13=w367:u16, element #14=w366:u16, element #15=w365:u16, element #16=w364:u16, element #17=w363:u16, element #18=w362:u16)
      n208 = Index Array(array=w245, index #1=w268, index #2=w269, index #3=w270, index #4=w271, index #5=w272, index #6=w273, index #7=w274, index #8=w275) -> (element #1=w330:u16, element #2=w328:u16, element #3=w327:u16, element #4=w326:u16, element #5=w325:u16, element #6=w324:u16, element #7=w323:u16, element #8=w322:u16)
      n209 = To Double Precision Float(number=w324) -> (double precision float=w321:dbl)
      n210 = To Double Precision Float(number=w323) -> (double precision float=w316:dbl)
      n211 = To Double Precision Float(number=w322) -> (double precision float=w315:dbl)
      n212 = Not Equal To 0?(x=w379) -> (x != 0?=w385:bool)
      n213 = Not Equal To 0?(x=w375) -> (x != 0?=w384:bool)
      n214 = Not Equal To 0?(x=w373) -> (x != 0?=w383:bool)
      n215 = Not Equal To 0?(x=w369) -> (x != 0?=w382:bool)
      n216 = Not Equal To 0?(x=w367) -> (x != 0?=w381:bool)
      n217 = Not Equal To 0?(x=w363) -> (x != 0?=w380:bool)
      n218 = Divide(x=w321, y=w317) -> (x/y=w320:dbl)
      n219 = Divide(x=w316, y=w317) -> (x/y=w319:dbl)
      n220 = Divide(x=w315, y=w317) -> (x/y=w318:dbl)
      n221 = local write "LC_Cue_First_OnOff"(w385) -> ()
      n222 = local write "LC_Cue_First_Block"(w378) -> ()
      n223 = local write "LC_Cue_First_Probability"(w377) -> ()
      n224 = local write "LC_Cue_First_Tdelay"(w376) -> ()
      n225 = local write "LC_Cue_First_delayOpt"(w384) -> ()
      n226 = local write "LC_Cue_First_Count"(w374) -> ()
      n227 = local write "LC_Cue_PreR_OnOff"(w383) -> ()
      n228 = local write "LC_Cue_PreR_Block"(w372) -> ()
      n229 = local write "LC_Cue_PreR_Probability"(w371) -> ()
      n230 = local write "LC_Cue_PreR_Tdelay"(w370) -> ()
      n231 = local write "LC_Cue_PreR_delayOpt"(w382) -> ()
      n232 = local write "LC_Cue_PreR_Count"(w368) -> ()
      n233 = local write "LC_Cue_PostR_OnOff"(w381) -> ()
      n234 = local write "LC_Cue_PostR_Block"(w366) -> ()
      n235 = local write "LC_Cue_PostR_Probability"(w365) -> ()
      n236 = local write "LC_Cue_PostR_Tdelay"(w364) -> ()
      n237 = local write "LC_Cue_PostR_delayOpt"(w380) -> ()
      n238 = local write "LC_Cue_PostR_Count"(w362) -> ()
      n239 = Not Equal To 0?(x=w330) -> (x != 0?=w329:bool)
      n240 = local write "LED_baseline"(w329) -> ()
      n241 = local write "Laser_Freq"(w328) -> ()
      n242 = local write "Laser_T"(w327) -> ()
      n243 = local write "Laser_Tpeak"(w326) -> ()
      n244 = local write "Laser_Tshutter"(w325) -> ()
      n245 = local write "Laser_power_min"(w320) -> ()
      n246 = local write "Laser_power_max"(w319) -> ()
      n247 = local write "Laser_power_step"(w318) -> ()
      n248 = call "BRig_dataLC_Selection_First_OnOff_l2.vi"() -> ("output_Selection_First_OnOff_l2"=w276:i32)  [unwired: 11 in]
      n249 = call "BRig_dataLC_Selection_First_Block_l2.vi"() -> ("output_Selection_First_Block_l2"=w277:i32)  [unwired: 11 in]
      n250 = call "BRig_dataLC_Selection_First_Prob_l2.vi"() -> ("output_Selection_First_Prob_l2"=w278:i32)  [unwired: 11 in]
      n251 = call "BRig_dataLC_Selection_First_Delay_l2.vi"() -> ("output_Selection_First_Delay_l2"=w279:i32)  [unwired: 11 in]
      n252 = call "BRig_dataLC_Selection_First_Count_l2.vi"() -> ("output_Selection_First_Count_l2"=w288:i32)  [unwired: 11 in]
      n253 = call "BRig_dataLC_Selection_PreR_OnOff_l2.vi"() -> ("output_Selection_PreR_OnOff_l2"=w280:i32)  [unwired: 11 in]
      n254 = call "BRig_dataLC_Selection_PreR_Block_l2.vi"() -> ("output_Selection_PreR_Block_l2"=w281:i32)  [unwired: 11 in]
      n255 = call "BRig_dataLC_Selection_PreR_Prob_l2.vi"() -> ("output_Selection_PreR_Prob_l2"=w282:i32)  [unwired: 11 in]
      n256 = call "BRig_dataLC_Selection_PreR_Delay_l2.vi"() -> ("output_Selection_PreR_Delay_l2"=w283:i32)  [unwired: 11 in]
      n257 = call "BRig_dataLC_Selection_PreR_Count_l2.vi"() -> ("output_Selection_PreR_Count_l2"=w289:i32)  [unwired: 11 in]
      n258 = call "BRig_dataLC_Selection_PostR_OnOff_l2.vi"() -> ("output_Selection_PostR_OnOff_l2"=w284:i32)  [unwired: 11 in]
      n259 = call "BRig_dataLC_Selection_PostR_Block_l2.vi"() -> ("output_Selection_PostR_Block_l2"=w285:i32)  [unwired: 11 in]
      n260 = call "BRig_dataLC_Selection_PostR_Prob_l2.vi"() -> ("output_Selection_PostR_Prob_l2"=w286:i32)  [unwired: 11 in]
      n261 = call "BRig_dataLC_Selection_PostR_Delay_l2.vi"() -> ("output_Selection_PostR_Delay_l2"=w287:i32)  [unwired: 11 in]
      n262 = call "BRig_dataLC_Selection_PostR_Count_l2.vi"() -> ("output_Selection_PostR_Count_l2"=w290:i32)  [unwired: 11 in]
      n263 = call "BRig_dataLC_Reward_OnOff_l2.vi"() -> ("output_Reward_OnOff_l2"=w258:i32)  [unwired: 11 in]
      n264 = call "BRig_dataLC_Reward_Block_l2.vi"() -> ("output_Reward_Block_l2"=w259:i32)  [unwired: 11 in]
      n265 = call "BRig_dataLC_Reward_Trial_l2.vi"() -> ("output_Reward_Trial_l2"=w260:i32)  [unwired: 11 in]
      n266 = call "BRig_dataLC_Reward_Prob_l2.vi"() -> ("output_Reward_Prob_l2"=w261:i32)  [unwired: 11 in]
      n267 = call "BRig_dataLC_Reward_Delay_l2.vi"() -> ("output_Reward_Delay_l2"=w266:i32)  [unwired: 11 in]
      n268 = call "BRig_dataLC_Wrong_OnOff_l2.vi"() -> ("output_Wrong_OnOff_l2"=w262:i32)  [unwired: 11 in]
      n269 = call "BRig_dataLC_Wrong_Block_l2.vi"() -> ("output_Wrong_Block_l2"=w263:i32)  [unwired: 11 in]
      n270 = call "BRig_dataLC_Wrong_Trial_l2.vi"() -> ("output_Wrong_Trial_l2"=w264:i32)  [unwired: 11 in]
      n271 = call "BRig_dataLC_Wrong_Prob_l2.vi"() -> ("output_Wrong_Prob_l2"=w265:i32)  [unwired: 11 in]
      n272 = call "BRig_dataLC_Wrong_Delay_l2.vi"() -> ("output_Wrong_Delay_l2"=w267:i32)  [unwired: 11 in]
      n273 = Index Array(array=w331, index #1=w258, index #2=w259, index #3=w260, index #4=w261, index #5=w266, index #6=w262, index #7=w263, index #8=w264, index #9=w265, index #10=w267) -> (element #1=w341:u16, element #2=w340:u16, element #3=w339:u16, element #4=w338:u16, element #5=w337:u16, element #6=w336:u16, element #7=w335:u16, element #8=w334:u16, element #9=w333:u16, element #10=w332:u16)
      n274 = Index Array(array=w331, index #1=w276, index #2=w277, index #3=w278, index #4=w279, index #5=w288, index #6=w280, index #7=w281, index #8=w282, index #9=w283, index #10=w289, index #11=w284, index #12=w285, index #13=w286, index #14=w287, index #15=w290) -> (element #1=w358:u16, element #2=w357:u16, element #3=w356:u16, element #4=w355:u16, element #5=w354:u16, element #6=w353:u16, element #7=w352:u16, element #8=w351:u16, element #9=w350:u16, element #10=w349:u16, element #11=w348:u16, element #12=w347:u16, element #13=w346:u16, element #14=w345:u16, element #15=w344:u16)
      n275 = Not Equal To 0?(x=w341) -> (x != 0?=w343:bool)
      n276 = Not Equal To 0?(x=w336) -> (x != 0?=w342:bool)
      n277 = Not Equal To 0?(x=w358) -> (x != 0?=w361:bool)
      n278 = Not Equal To 0?(x=w353) -> (x != 0?=w360:bool)
      n279 = Not Equal To 0?(x=w348) -> (x != 0?=w359:bool)
      n280 = local write "LC_Reward_OnOff"(w343) -> ()
      n281 = local write "LC_Reward_Block"(w340) -> ()
      n282 = local write "LC_Reward_Trial"(w339) -> ()
      n283 = local write "LC_Reward_Probability"(w338) -> ()
      n284 = local write "LC_Reward_Tdelay"(w337) -> ()
      n285 = local write "LC_Wrong_OnOff"(w342) -> ()
      n286 = local write "LC_Wrong_Block"(w335) -> ()
      n287 = local write "LC_Wrong_Trial"(w334) -> ()
      n288 = local write "LC_Wrong_Probability"(w333) -> ()
      n289 = local write "LC_Wrong_Tdelay"(w332) -> ()
      n290 = local write "LC_Sel_First_OnOff"(w361) -> ()
      n291 = local write "LC_Sel_First_Block"(w357) -> ()
      n292 = local write "LC_Sel_First_Probability"(w356) -> ()
      n293 = local write "LC_Sel_First_Tdelay"(w355) -> ()
      n294 = local write "LC_Sel_First_Count"(w354) -> ()
      n295 = local write "LC_Sel_PreR_OnOff"(w360) -> ()
      n296 = local write "LC_Sel_PreR_Block"(w352) -> ()
      n297 = local write "LC_Sel_PreR_Probability"(w351) -> ()
      n298 = local write "LC_Sel_PreR_Tdelay"(w350) -> ()
      n299 = local write "LC_Sel_PreR_Count"(w349) -> ()
      n300 = local write "LC_Sel_PostR_OnOff"(w359) -> ()
      n301 = local write "LC_Sel_PostR_Block"(w347) -> ()
      n302 = local write "LC_Sel_PostR_Probability"(w346) -> ()
      n303 = local write "LC_Sel_PostR_Tdelay"(w345) -> ()
      n304 = local write "LC_Sel_PostR_Count"(w344) -> ()
    }
  }
  "output_dataLC" <- w4
  "output_dataExp" <- w1
